vi "Logging module-status updater.vi"(8 "error in":errorcluster, 9 "Queue element":T1 {"Ref Dwell time (us)" format="%#.6g"; "Frame Size" items=["100X100"=100, "128X128"=128, "200X200"=200, "256X256"=256, "512X512"=512, "1024x1024"=1024, "2048x2048"=2048]; "Dwell time (us)" format="%#.6g"}, 11 "Message Queues":T5) -> (0 "error out":errorcluster)   [LabVIEW 2020]
uses:
  User Interface/Queue/Message Queue/Typedefs/All Message Queues.ctl
  User Interface/Queue/Message Queue/Typedefs/Message Cluster.ctl
  Typedefs/Logging queue element.ctl
  Typedefs/Imaging Protocols enum.ctl
  Typedefs/Frame Size.ctl
  Typedefs/Acquired points count.ctl
  Global Variables/General Globals.vi
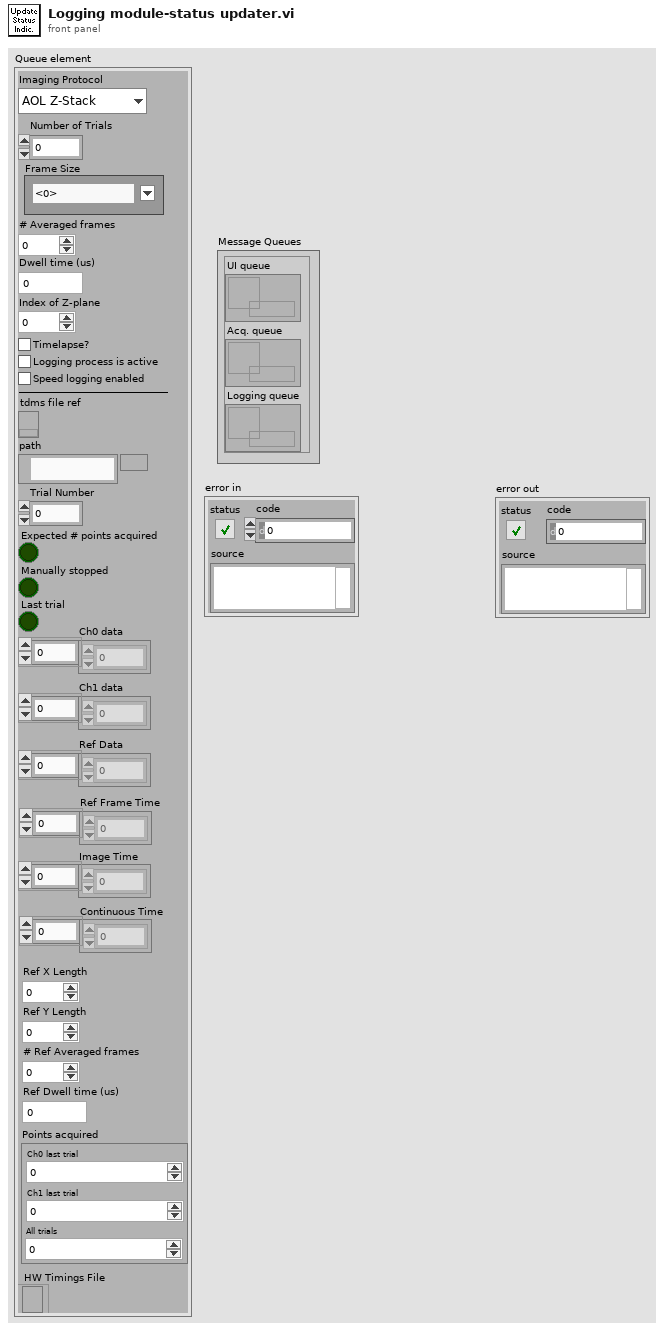
[diagram p1: front panel]
types:
  T1 = typedef "Logging queue element.ctl" = cluster{"Imaging Protocol":T2, "Number of Trials":u16, "Frame Size":T3, "# Averaged frames":u16, "Dwell time (us)":dbl, "Index of Z-plane":i32, "Timelapse?":bool, "Logging process is active":bool, "Speed logging enabled":bool, "tdms file ref":refnum<k34>, "path":path, "Trial Number":i32, "Expected # points acquired":bool, "Manually stopped":bool, "Last trial":bool, "Ch0 data":u32[], "Ch1 data":u32[], "Ref Data":u32[], "Ref Frame Time":u64[], "Image Time":u64[], "Continuous Time":u64[], "Ref X Length":u16, "Ref Y Length":u16, "# Ref Averaged frames":u16, "Ref Dwell time (us)":dbl, "Points acquired":T4, "HW Timings File":refnum<file>}
  T2 = typedef "Imaging Protocols enum.ctl" = enum16{"AOL Z-Stack", "Motor Z Stack", "Functional Acquisition", "Single Plane Acquisition", "Volume Acquisition", "Live Imaging", "Live Plane Imaging", "Live Volume Imaging"}
  T3 = typedef "Frame Size.ctl" = u16
  T4 = typedef "Acquired points count.ctl" = cluster{"Ch0 last trial":u64, "Ch1 last trial":u64, "All trials":u64}
  T5 = typedef "All Message Queues.ctl" = cluster{"UI queue":refnum<queue>, "Acq. queue":refnum<queue>, "Logging queue":refnum<queue>}
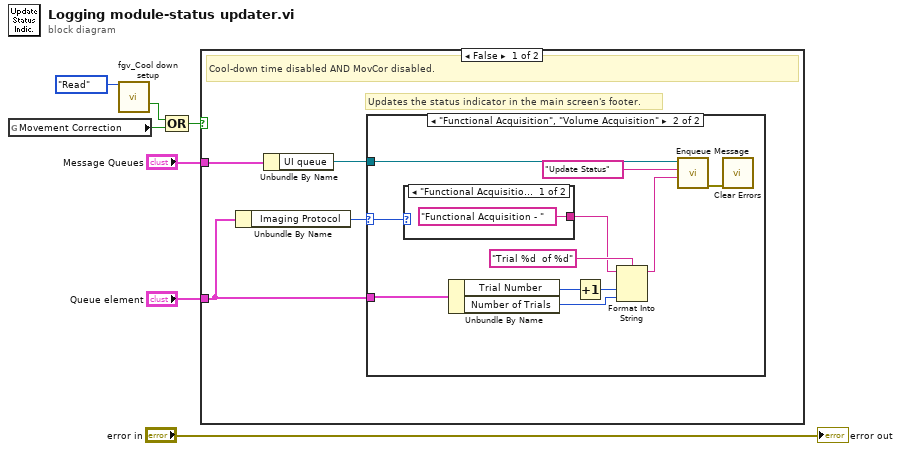
[diagram p0: block diagram]
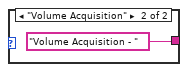
[diagram p3: hidden frame]
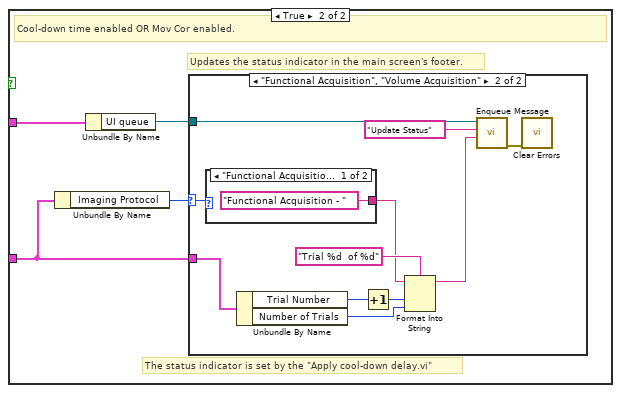
[diagram p4: hidden frame]
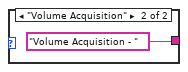
[diagram p6: hidden frame]
diagram:
  n1 = global read "General Globals.vi" "Movement Correction"() -> (w3:bool)
  n2 = call "fgv_Cool down setup.vi"("Function"=enum16{"Intialize", "Write", "Read", "Clear"}."Read") -> ("Enable cool-down time"=w2:bool)  [unwired: 12 in, 2 out]
  n3 = Compound Arithmetic op=OR(w2, w3) -> (w1:bool)
  n4 = case shown="False" w1 {
    tunnel: "Message Queues" -> [w11 w25]
    tunnel: "Queue element" -> [w9 w26]
    frame False {
      # "Updates the status indicator in the main screen's footer."
      # "Cool-down time disabled AND MovCor disabled."
      n5 = Unbundle By Name(w9) -> ("Imaging Protocol"=w8:T2)
      n6 = Unbundle By Name(w11) -> ("UI queue"=w10:refnum<queue>)
      n7 = case shown="\"Functional Acquisition\", \"Volume Acquisition\"" w8 {
        selector: w8 -> [_ w13]
        tunnel: w10 -> [_ w20]
        tunnel: w9 -> [_ w14]
        frame Default {
        }
        frame "Functional Acquisition", "Volume Acquisition" {
          n8 = case shown="\"Functional Acquisition\", Default" w13 {
            tunnel: ["Functional Acquisition - " "Volume Acquisition - "] -> w15
            frame "Functional Acquisition", Default {
            }
            frame "Volume Acquisition" {
            }
          }
          n9 = Unbundle By Name(w14) -> ("Trial Number"=w18:i32, "Number of Trials"=w16:u16)
          n10 = Increment(x=w18) -> (x+1=w17:i32)
          n11 = Format Into String(format string="Trial %d  of %d" ("Acquiring and Logging..."), initial string=w15, w17, w16) -> (resulting string=w12:string)  [unwired: 1 in, 1 out]
          n12 = call "Enqueue Message.vi"("Message Data"=w12, "Message"="Update Status", "Queue"=w20) -> ("error out"=w21:errorcluster)  [unwired: 7 in, 1 out]
          n13 = call <vilib>:"Clear Errors.vi"("error in (no error)"=w21) -> ()  [unwired: 5 in, 2 out]
        }
      }
    }
    frame True {
      # "Updates the status indicator in the main screen's footer."
      # "The status indicator is set by the \"Apply cool-down delay.vi\""
      # "Cool-down time enabled OR Mov Cor enabled."
      n14 = Unbundle By Name(w26) -> ("Imaging Protocol"=w27:T2)
      n15 = Unbundle By Name(w25) -> ("UI queue"=w28:refnum<queue>)
      n16 = case shown="\"Functional Acquisition\", \"Volume Acquisition\"" w27 {
        selector: w27 -> [_ w31]
        tunnel: w28 -> [_ w37]
        tunnel: w26 -> [_ w33]
        frame Default {
        }
        frame "Functional Acquisition", "Volume Acquisition" {
          n17 = case shown="\"Functional Acquisition\", Default" w31 {
            tunnel: ["Functional Acquisition - " "Volume Acquisition - "] -> w29
            frame "Functional Acquisition", Default {
            }
            frame "Volume Acquisition" {
            }
          }
          n18 = Unbundle By Name(w33) -> ("Trial Number"=w34:i32, "Number of Trials"=w30:u16)
          n19 = Increment(x=w34) -> (x+1=w32:i32)
          n20 = Format Into String(format string="Trial %d  of %d" ("Acquiring and Logging..."), initial string=w29, w32, w30) -> (resulting string=w35:string)  [unwired: 1 in, 1 out]
          n21 = call "Enqueue Message.vi"("Message Data"=w35, "Message"="Update Status", "Queue"=w37) -> ("error out"=w38:errorcluster)  [unwired: 7 in, 1 out]
          n22 = call <vilib>:"Clear Errors.vi"("error in (no error)"=w38) -> ()  [unwired: 5 in, 2 out]
        }
      }
    }
  }
  "error out" <- "error in"
